vi "XY_dispense.vi"(0 "Vacuum Setting (0000)":i64=20, 1 "Pressure":i16=20, 6 "Speed":dbl=20.0 format="%#_13g", 8 "axis names":string[](array[string])=["Y"], 9 "distances":dbl[](array[numeric])=[230.0], 10 "Ultimus V in":refnum<class "Ultimus V2.lvclass">, 11 "Motion in":refnum<class "Motion.lvclass">) -> (2 "Ultimus V out":refnum<class "Ultimus V2.lvclass">, 3 "Motion out":refnum<class "Motion.lvclass">)   [LabVIEW 2016]
uses:
  Classes/Controllers/Motion/Copy of Motion Folder/Motion.lvclass
  Classes/Controllers/Dispenser/Copy of Ultimus V2 Folder/Ultimus V2.lvclass
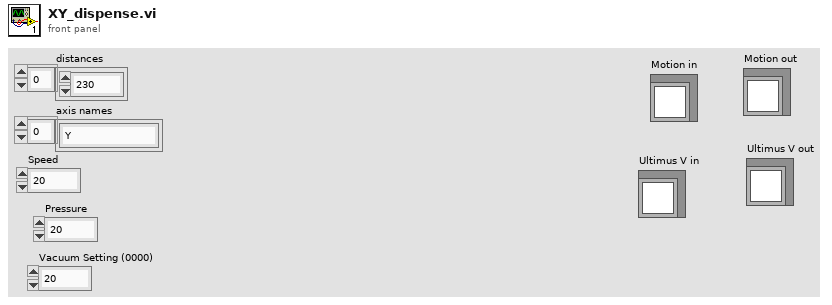
[diagram p1: front panel]
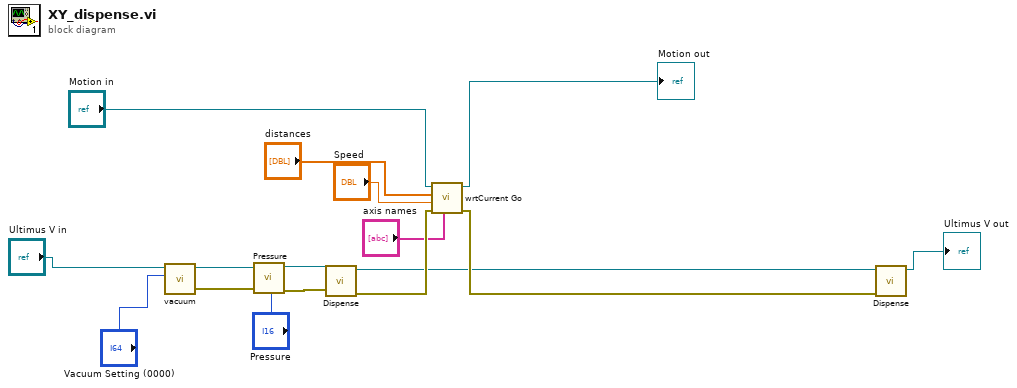
[diagram p0: block diagram]
diagram:
  n1 = call "vacuum.vi"("Vacuum Setting (0000)"="Vacuum Setting (0000)", "Ultimus V in"="Ultimus V in") -> ("error out"=w12:errorcluster, "Ultimus V out"=w15:refnum<class "Ultimus V2.lvclass">)  [unwired: 8 in]
  n2 = call-dynamic "Pressure.vi"("error in (no error)"=w12, "Pressure"="Pressure", "Ultimus V in"=w15) -> ("error out"=w11:errorcluster, "Ultimus V out"=w16:refnum<class "Ultimus V2.lvclass">)  [unwired: 7 in]
  n3 = call-dynamic "Dispense.vi"("error in (no error)"=w11, "Ultimus V in"=w16) -> ("error out"=w8:errorcluster, "Ultimus V out"=w6:refnum<class "Ultimus V2.lvclass">)  [unwired: 8 in]
  n4 = call-dynamic "wrtCurrent Go.vi"("axis names"="axis names", "error in (no error)"=w8, "Speed"="Speed", "distances"="distances", "Motion in"="Motion in") -> ("error out"=w7:errorcluster, "Motion out"=→"Motion out":refnum<class "Motion.lvclass">)  [unwired: 5 in]
  n5 = call-dynamic "Dispense.vi"("error in (no error)"=w7, "Ultimus V in"=w6) -> ("Ultimus V out"=→"Ultimus V out":refnum<class "Ultimus V2.lvclass">)  [unwired: 8 in, 1 out]
